vi "VariableToCluster.vi"(11 "Variable":refnum<class "Variable.lvclass">) -> (3 "VariableCluster":T1)   [LabVIEW 2012, in "VariableManagerAPI.lvlib"]
uses:
  VariableManagerAPI.lvlib
  Variable/Variable.lvclass
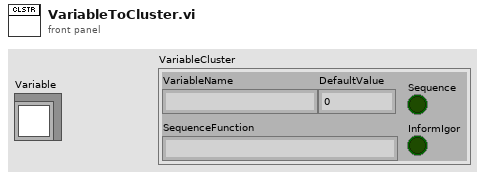
[diagram p1: front panel]
types:
  T1 = cluster{"VariableName":string, "DefaultValue":dbl, "SequenceFunction":string, "Sequence":bool, "InformIgor":bool}
  T2 = cluster{"Accessors:VariableName":string, "Accessors:DefaultValue":dbl, "Accessors:SequenceFunction":string, "Accessors:Sequence":bool, "Accessors:InformIgor":bool}
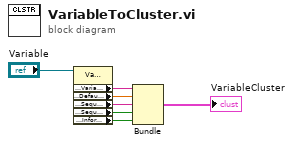
[diagram p0: block diagram]
diagram:
  n1 = property class="Variable.lvclass"(reference="Variable") -> ("Accessors:VariableName"=w6:string, "Accessors:DefaultValue"=w5:dbl, "Accessors:SequenceFunction"=w4:string, "Accessors:Sequence"=w3:bool, "Accessors:InformIgor"=w2:bool)  [unwired: 1 in, 2 out]
  n2 = Bundle("Accessors:VariableName"=w6, "Accessors:DefaultValue"=w5, "Accessors:SequenceFunction"=w4, "Accessors:Sequence"=w3, "Accessors:InformIgor"=w2) -> (→"VariableCluster":T2)  [unwired: 1 in]
